vi "加标回收启动对话框.vi"(11 "测试模式":enum16{"水样测试", "平行样测试", "加标回收", "集成干预测试"}(ring)) -> (1 "流程参数":T1, 2 "启动参数":T2, 3 "check ？":bool)   [LabVIEW 2016, in "质控单元V4.lvlib"]
panel:
  in  "采配水":bool=TRUE
  in  "取消":bool
  in  "确认":bool
  in  "CODCr":bool caption="启用"
  in  "CODMn":bool caption="启用"
  in  "总氮":bool caption="启用"
  in  "总磷":bool caption="启用"
  in  "氨氮":bool caption="启用"
  # "请选择启动参数和流程"
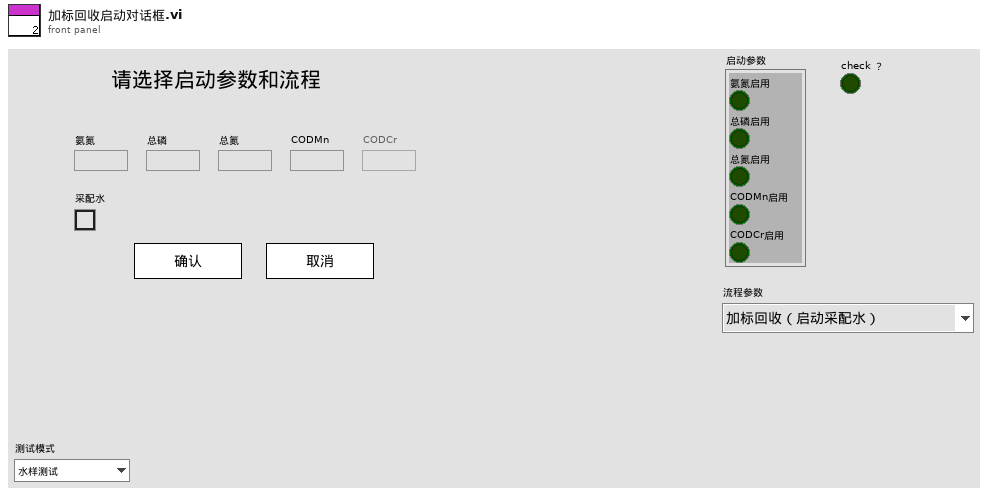
[diagram p1: front panel]
types:
  T1 = typedef "质控单元V4.lvlib/测试流程.ctl" = enum16{"加标回收（启动采配水）", "加标回收（不启动采配水）", "水样测试（启动采配水）", "水样测试（不启动采配水）", "平行样测试（启动采配水）", "平行样测试（不启动采配水）", "集成干预测试"}
  T2 = cluster{"氨氮启用":bool, "总磷启用":bool, "总氮启用":bool, "CODMn启用":bool, "CODCr启用":bool}
  T3 = cluster{"氨氮":bool, "总磷":bool, "总氮":bool, "CODMn":bool, "CODCr":bool}
  T4 = cluster{"氨氮":bool, "总磷":bool, "总氮":bool, "CODMn":bool, "CODCr":bool, "氨氮总磷":bool, "总磷总氮":bool}
  T5 = enum8{"Enabled", "Disabled", "Disabled and Grayed Out"}
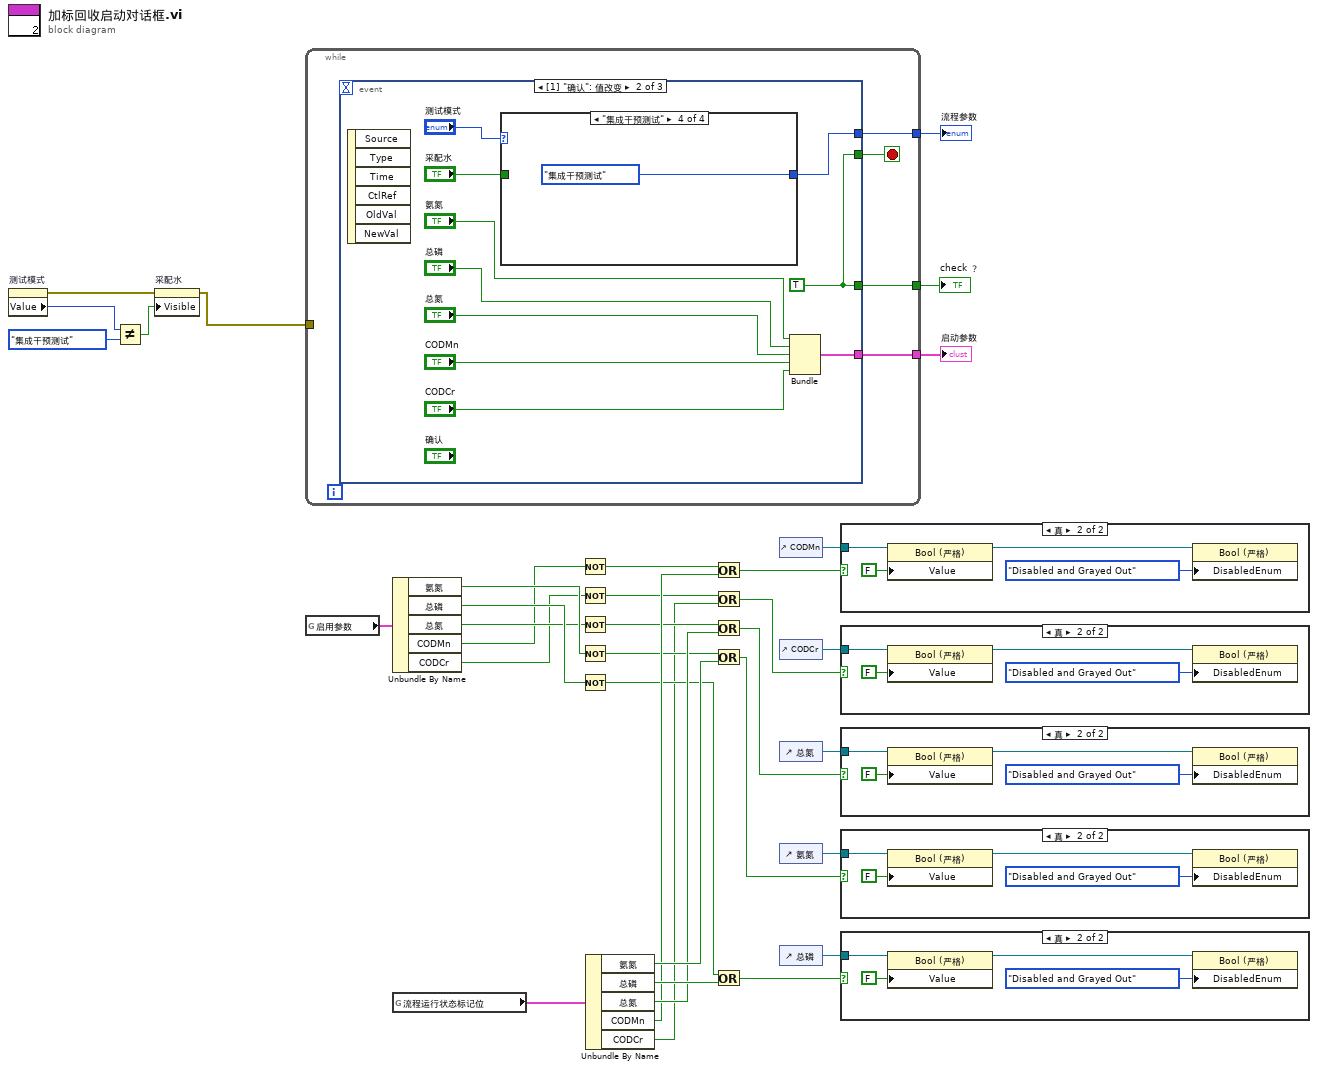
[diagram p0: block diagram]
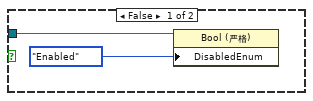
[diagram p2: hidden frame]
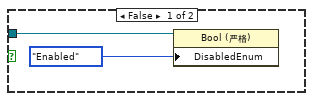
[diagram p3: hidden frame]
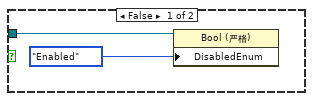
[diagram p4: hidden frame]
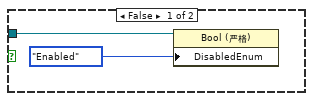
[diagram p5: hidden frame]
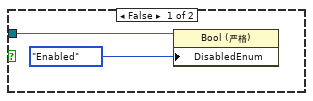
[diagram p6: hidden frame]
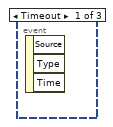
[diagram p7: hidden frame]
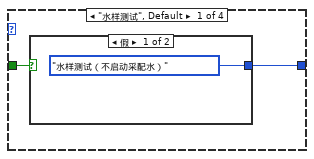
[diagram p8: hidden frame]
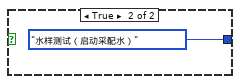
[diagram p9: hidden frame]
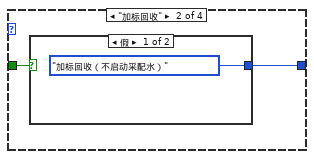
[diagram p10: hidden frame]
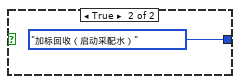
[diagram p11: hidden frame]
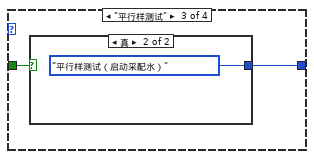
[diagram p12: hidden frame]
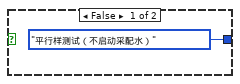
[diagram p13: hidden frame]
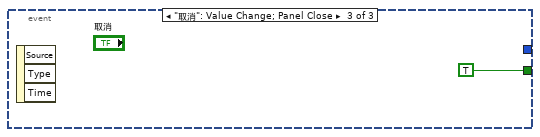
[diagram p14: hidden frame]
diagram:
  n1 = property on="测试模式" class="Enum (严格)"() -> (error out=w3:errorcluster, "Value"=w5:enum16{"水样测试", "平行样测试", "加标回收", "集成干预测试"})  [unwired: 2 in, 1 out]
  n2 = Not Equal?(x=w5, y=enum16{"水样测试", "平行样测试", "加标回收", "集成干预测试"}."集成干预测试") -> (x != y?=w2:bool)
  n3 = property on="采配水" class="Bool (严格)"(error in=w3, "Visible"=w2) -> (error out=w1:errorcluster)  [unwired: 1 in, 1 out]
  n4 = while {
    tunnel: [w39] -> w35
    tunnel: [w37] -> w34
    tunnel: [w36] -> w33
    tunnel: w1 -> [_]
    stop <- w38 stop-if-true
    n5 = event shown="[1] \"确认\": 值改变" {
      selector: _ -> [_ _ _]
      dyn-events: _ -> [_ _ _]
      timeout: _ -> [_ _ _]
      tunnel: [_ w49 _] -> w39
      tunnel: [_ w49 TRUE] -> w38
      tunnel: [_ w43 _] -> w37
      tunnel: [_ w41 _] -> w36
      event Timeout {
        n6 = event-data() -> ()  [unwired: 1 in, 3 out]
      }
      event "确认": Value Change {
        w49 = TRUE
        n7 = event-data() -> ()  [unwired: 1 in, 6 out]
        n8 = case shown="\"集成干预测试\"" "测试模式" {
          tunnel: "采配水" -> [w51 w55 w59 _]
          tunnel: [w50 w54 w58 测试流程."集成干预测试" ("流程")] -> w41
          frame "水样测试", Default {
            n9 = case shown="假" w51 {
              tunnel: [测试流程."水样测试（不启动采配水）" ("流程") 测试流程."水样测试（启动采配水）" ("流程")] -> w50
              frame False {
              }
              frame True {
              }
            }
          }
          frame "加标回收" {
            n10 = case shown="假" w55 {
              tunnel: [测试流程."加标回收（不启动采配水）" ("流程") 测试流程."加标回收（启动采配水）" ("流程")] -> w54
              frame False {
              }
              frame True {
              }
            }
          }
          frame "平行样测试" {
            n11 = case shown="真" w59 {
              tunnel: [测试流程."平行样测试（不启动采配水）" ("流程") 测试流程."平行样测试（启动采配水）" ("流程")] -> w58
              frame False {
              }
              frame True {
              }
            }
          }
          frame "集成干预测试" {
          }
        }
        n12 = Bundle("氨氮"="氨氮", "总磷"="总磷", "总氮"="总氮", "CODMn"="CODMn", "CODCr"="CODCr") -> (w43:T3)  [unwired: 1 in]
      }
      event "取消": Value Change; Panel Close {
        n13 = event-data() -> ()  [unwired: 1 in, 3 out]
      }
    }
  }
  "check ？" <- w35
  "启动参数" <- w34
  "流程参数" <- w33
  n14 = global read "ZK断电保存全局变量.vi" "启用参数"() -> (w22:T4)
  n15 = Unbundle By Name(w22) -> ("氨氮"=w17:bool, "总磷"=w20:bool, "总氮"=w14:bool, "CODMn"=w10:bool, "CODCr"=w8:bool)
  n16 = global read "ZK非断电保存全局变量.vi" "流程运行状态标记位"() -> (w32:T3)
  n17 = Not(x=w10) -> (.not. x?=w11:bool)
  n18 = Not(x=w8) -> (.not. x?=w9:bool)
  n19 = Not(x=w14) -> (.not. x?=w13:bool)
  n20 = Not(x=w17) -> (.not. x?=w16:bool)
  n21 = Not(x=w20) -> (.not. x?=w19:bool)
  n22 = Unbundle By Name(w32) -> ("氨氮"=w31:bool, "总磷"=w28:bool, "总氮"=w26:bool, "CODMn"=w24:bool, "CODCr"=w7:bool)
  n23 = Or(x=w11, y=w24) -> (x .or. y?=w12:bool)
  n24 = Or(x=w9, y=w7) -> (x .or. y?=w6:bool)
  n25 = Or(x=w13, y=w26) -> (x .or. y?=w15:bool)
  n26 = Or(x=w16, y=w31) -> (x .or. y?=w18:bool)
  n27 = Or(x=w19, y=w28) -> (x .or. y?=w21:bool)
  n28 = control-ref of="CODMn"() -> (w25:refnum<vi>)
  n29 = control-ref of="CODCr"() -> (w23:refnum<vi>)
  n30 = control-ref of="总氮"() -> (w27:refnum<vi>)
  n31 = control-ref of="氨氮"() -> (w30:refnum<vi>)
  n32 = control-ref of="总磷"() -> (w29:refnum<vi>)
  n33 = case shown="真" w12 {
    tunnel: w25 -> [w64 w69]
    frame False {
      n34 = property class="Bool (严格)"(reference=w64, "DisabledEnum"=T5."Enabled" ("禁用")) -> ()  [unwired: 1 in, 2 out]
    }
    frame True {
      n35 = property class="Bool (严格)"(reference=w69, "Value"=FALSE ("值")) -> (reference out=w67:refnum<vi>)  [unwired: 1 in, 1 out]
      n36 = property class="Bool (严格)"(reference=w67, "DisabledEnum"=T5."Disabled and Grayed Out" ("禁用")) -> ()  [unwired: 1 in, 2 out]
    }
  }
  n37 = case shown="真" w6 {
    tunnel: w23 -> [w70 w75]
    frame False {
      n38 = property class="Bool (严格)"(reference=w70, "DisabledEnum"=T5."Enabled" ("禁用")) -> ()  [unwired: 1 in, 2 out]
    }
    frame True {
      n39 = property class="Bool (严格)"(reference=w75, "Value"=FALSE ("值")) -> (reference out=w73:refnum<vi>)  [unwired: 1 in, 1 out]
      n40 = property class="Bool (严格)"(reference=w73, "DisabledEnum"=T5."Disabled and Grayed Out" ("禁用")) -> ()  [unwired: 1 in, 2 out]
    }
  }
  n41 = case shown="真" w15 {
    tunnel: w27 -> [w76 w81]
    frame False {
      n42 = property class="Bool (严格)"(reference=w76, "DisabledEnum"=T5."Enabled" ("禁用")) -> ()  [unwired: 1 in, 2 out]
    }
    frame True {
      n43 = property class="Bool (严格)"(reference=w81, "Value"=FALSE ("值")) -> (reference out=w79:refnum<vi>)  [unwired: 1 in, 1 out]
      n44 = property class="Bool (严格)"(reference=w79, "DisabledEnum"=T5."Disabled and Grayed Out" ("禁用")) -> ()  [unwired: 1 in, 2 out]
    }
  }
  n45 = case shown="真" w18 {
    tunnel: w30 -> [w82 w87]
    frame False {
      n46 = property class="Bool (严格)"(reference=w82, "DisabledEnum"=T5."Enabled" ("禁用")) -> ()  [unwired: 1 in, 2 out]
    }
    frame True {
      n47 = property class="Bool (严格)"(reference=w87, "Value"=FALSE ("值")) -> (reference out=w85:refnum<vi>)  [unwired: 1 in, 1 out]
      n48 = property class="Bool (严格)"(reference=w85, "DisabledEnum"=T5."Disabled and Grayed Out" ("禁用")) -> ()  [unwired: 1 in, 2 out]
    }
  }
  n49 = case shown="真" w21 {
    tunnel: w29 -> [w88 w93]
    frame False {
      n50 = property class="Bool (严格)"(reference=w88, "DisabledEnum"=T5."Enabled" ("禁用")) -> ()  [unwired: 1 in, 2 out]
    }
    frame True {
      n51 = property class="Bool (严格)"(reference=w93, "Value"=FALSE ("值")) -> (reference out=w91:refnum<vi>)  [unwired: 1 in, 1 out]
      n52 = property class="Bool (严格)"(reference=w91, "DisabledEnum"=T5."Disabled and Grayed Out" ("禁用")) -> ()  [unwired: 1 in, 2 out]
    }
  }
